vi "Measure.vi"(6 "Graph in":cluster{dbl[], dbl[]}, 7 "XY Graph":refnum<vi>, 8 "error in":errorcluster, 10 "Reference Cell":i32) -> (0 "error out":errorcluster, 1 "Values":cluster{dbl[], dbl[]}, 2 "P1/P2":dbl format="%#_13g")   [LabVIEW 2013]
uses:
  <vilib>/Analysis/baseanly.llb/Mean (DBL).vi
  <vilib>/Analysis/NI_AALBase.lvlib
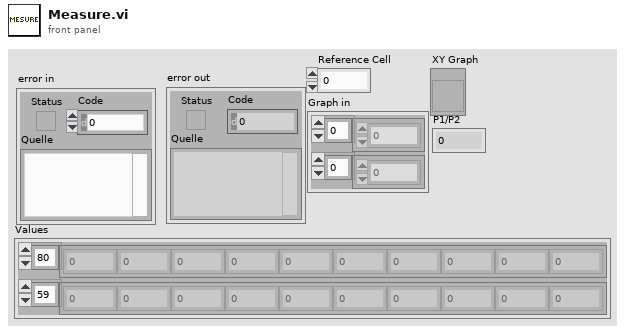
[diagram p1: front panel]
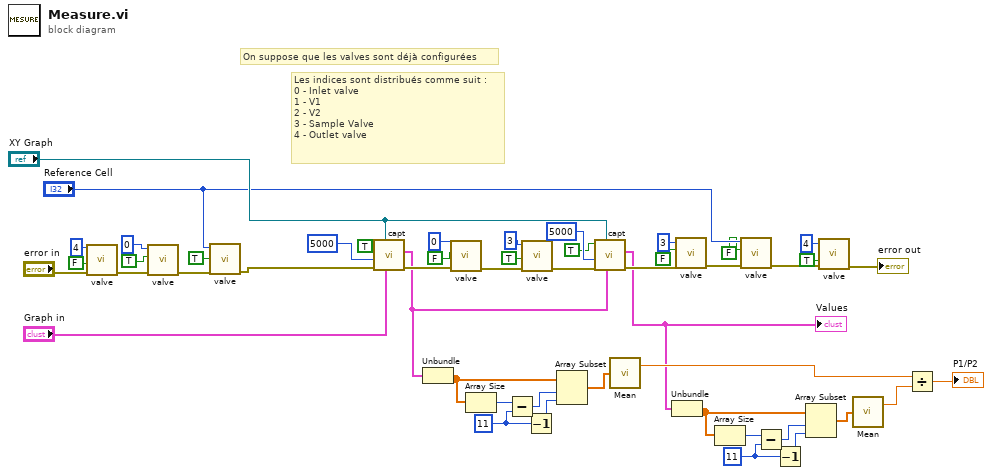
[diagram p0: block diagram]
diagram:
  w3 = 11
  w8 = 11
  # "On suppose que les valves sont déjà configurées"
  # "Les indices sont distribués comme suit :\n0 - Inlet valve\n1 - V1\n2 - V2\n3 - Sample Valve\n4 - Outlet valve"
  n1 = call "valve.vi"("error in"="error in", "ON"=FALSE, "Valve"=4) -> ("error out"=w39:errorcluster)  [unwired: 8 in]
  n2 = call "valve.vi"("error in"=w39, "ON"=TRUE, "Valve"=0) -> ("error out"=w35:errorcluster)  [unwired: 8 in]
  n3 = call "valve.vi"("error in"=w35, "ON"=TRUE, "Valve"="Reference Cell") -> ("error out"=w34:errorcluster)  [unwired: 8 in]
  n4 = call "capt.vi"("Graph in"="Graph in", "XY Graph"="XY Graph", "error in"=w34, "Length"=5000, "ON"=TRUE) -> ("error out"=w45:errorcluster, "Values"=w14:cluster{dbl[], dbl[]})  [unwired: 5 in]
  n5 = Unbundle(w14) -> (w12:dbl[])  [unwired: 1 out]
  n6 = call "valve.vi"("error in"=w45, "ON"=FALSE, "Valve"=0) -> ("error out"=w32:errorcluster)  [unwired: 8 in]
  n7 = Array Size(array=w12) -> (size(s)=w11:i32)
  n8 = Subtract(x=w11, y=w8) -> (x-y=w10:i32)
  n9 = call "valve.vi"("error in"=w32, "ON"=TRUE, "Valve"=3) -> ("error out"=w28:errorcluster)  [unwired: 8 in]
  n10 = Decrement(x=w8) -> (x-1=w9:i32)
  n11 = Array Subset(array=w12, index=w10, length=w9) -> (w13:dbl[])
  n12 = call "capt.vi"("Graph in"=w14, "XY Graph"="XY Graph", "error in"=w28, "Length"=5000, "ON"=TRUE) -> ("error out"=w24:errorcluster, "Values"=w2:cluster{dbl[], dbl[]})  [unwired: 5 in]
  "Values" <- w2
  n13 = call-poly <vilib>:"Mean.vi"("X"=w13) -> ("mean"=w17:dbl)  [unwired: 1 out]
  n14 = Unbundle(w2) -> (w7:dbl[])  [unwired: 1 out]
  n15 = call "valve.vi"("error in"=w24, "ON"=FALSE, "Valve"=3) -> ("error out"=w23:errorcluster)  [unwired: 8 in]
  n16 = Array Size(array=w7) -> (size(s)=w6:i32)
  n17 = call "valve.vi"("error in"=w23, "ON"=FALSE, "Valve"="Reference Cell") -> ("error out"=w22:errorcluster)  [unwired: 8 in]
  n18 = Subtract(x=w6, y=w3) -> (x-y=w5:i32)
  n19 = Decrement(x=w3) -> (x-1=w4:i32)
  n20 = Array Subset(array=w7, index=w5, length=w4) -> (w1:dbl[])
  n21 = call "valve.vi"("error in"=w22, "ON"=TRUE, "Valve"=4) -> ("error out"=→"error out":errorcluster)  [unwired: 8 in]
  n22 = call-poly <vilib>:"Mean.vi"("X"=w1) -> ("mean"=w16:dbl)  [unwired: 1 out]
  n23 = Divide(x=w17, y=w16) -> (x/y=→"P1/P2":dbl)
